vi "NI VeriStand - Start Multiple Waveforms Multi t0 (CDB).vi"(8 "error in (no error)":errorcluster, 10 "t0s":timestamp[](array[timestamp]), 11 "Multiple Waveforms Write Session (CDB) in":refnum<class "Multiple Waveforms Write (CDB).lvclass">) -> (0 "error out":errorcluster, 3 "Multiple Waveforms Write Session (CDB) out":refnum<class "Multiple Waveforms Write (CDB).lvclass">)   [LabVIEW 2020, in "NI_VS Custom Device Waveform API.lvlib" / "Multiple Waveforms Write (CDB).lvclass"]
doc: "Sets the start time (t0) for the waveform data you want to write with the Write Waveform(s) VI. NI VeriStand considers all data the custom device writes to a waveform be continuous unless this VI executes again with a different start time."
uses:
  Multiple Waveforms Write (CDB).lvclass
  D:/p4/penguin/lvaddon/Veristand/master/src/LabVIEW/vilib/NI VeriStand/Custom Device Waveform API/Waveform Session.lvclass
  Waveform Session.lvclass/Waveform Session.ctl
  Multiple Waveforms Write (CDB).lvclass/Multiple Waveforms Write (CDB).ctl
  Internal Comm Classes/WPL Comm/WPL Comm.lvclass/WPL Comm.ctl
  Internal Comm Classes/WPL Comm/Send WPL Command.vi
  Internal Comm Classes/WPL Comm/Set Multi t0 on Variant.vi
  Internal Comm Classes/WPL Comm/Convert Q Error to Shutdown Error.vi
  Internal Comm Classes/WPL Comm/WPL Comm (2D CDB)/WPL Comm (2D CDB).lvclass
  D:/p4/penguin/lvaddon/Veristand/master/src/LabVIEW/vilib/NI VeriStand/Custom Device Waveform API/Internal Comm Classes/WPL Comm/WPL Comm.lvclass
  <vilib>/Utility/error.llb/Error Cluster From Error Code.vi
  Waveform Session.lvclass
  Internal Comm Classes/WPL Comm/WPL Comm.lvclass
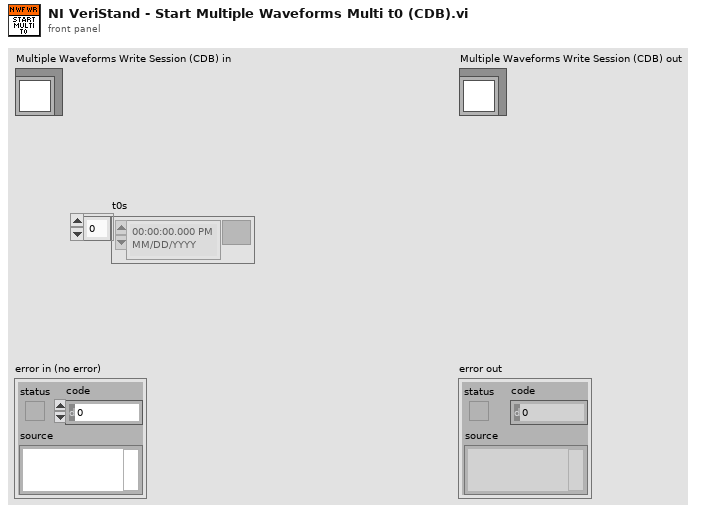
[diagram p1: front panel]
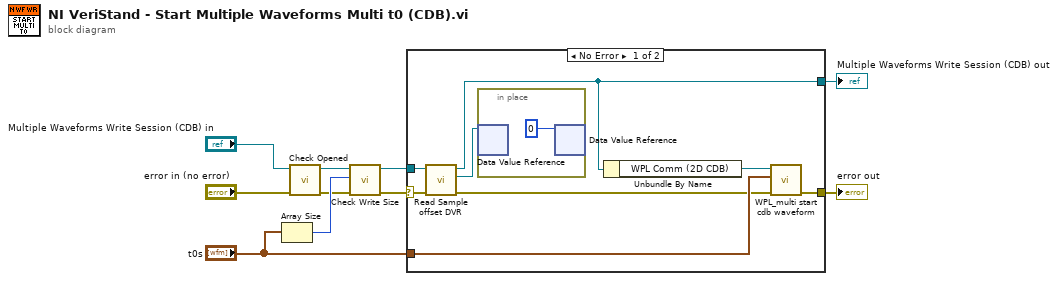
[diagram p0: block diagram]
diagram:
  n1 = Array Size(array="t0s") -> (size(s)=w6:i32)
  n2 = call "Check Opened.vi"("error in (no error)"="error in (no error)", "Waveform Session in"="Multiple Waveforms Write Session (CDB) in") -> ("error out"=w3:errorcluster, "Waveform Session out"=w5:refnum<class "Multiple Waveforms Write (CDB).lvclass">)  [unwired: 8 in]
  n3 = call "Check Write Size.vi"("error in (no error)"=w3, "# Of Waveforms"=w6, "Waveform Session in"=w5) -> ("error out"=w2:errorcluster, "Waveform Session out"=w4:refnum<class "Multiple Waveforms Write (CDB).lvclass">)  [unwired: 7 in]
  n4 = case shown="No Error" w2 {
    selector: w2 -> [w11 w20]
    tunnel: [w16 w20] -> w10
    tunnel: [w12 w19] -> w9
    tunnel: w4 -> [w13 w19]
    tunnel: "t0s" -> [w15 _]
    frame No Error {
      n5 = call "Read Sample offset DVR.vi"("Waveform Session in"=w13) -> ("Sample offset"=w14:refnum<data-value>, "Waveform Session out"=w12:refnum<class "Multiple Waveforms Write (CDB).lvclass">)  [unwired: 9 in]
      n6 = in-place {
        n7 = in-place-dvr #1(w14) -> ()  [unwired: 2 out]
        n8 = in-place-dvr #1(u64 0 ("data value")) -> ()  [unwired: 2 out]
      }
      n9 = Unbundle By Name(w12) -> ("WPL Comm (2D CDB)"=w17:refnum<class "WPL Comm (2D CDB).lvclass">)
      n10 = call "WPL_multi start cdb waveform.vi"("error in (no error)"=w11, "t0s"=w15, "WPL Comm in"=w17) -> ("error out"=w16:errorcluster)  [unwired: 8 in]
    }
    frame Error {
    }
  }
  "error out" <- w10
  "Multiple Waveforms Write Session (CDB) out" <- w9
